vi "State_Machine.vi"(8 "error in (no error)":errorcluster caption="entrée d'erreur (pas d'erreur)", 11 "Get_Voltage en entrée":refnum<class "Zigbee_Reset.lvclass">) -> (0 "error out":errorcluster caption="sortie d'erreur", 2 "Json_String":string, 3 "Get_Voltage en sortie":refnum<class "Zigbee_Reset.lvclass">)   [LabVIEW 2020, in "Library Test.lvlib" / "Zigbee_Reset.lvclass"]
uses:
  Zigbee_Reset.lvclass
  C:/Users/ngarcin/OneDrive - Altyor/Standard TB/Class/Test/Zigbee_Send_Command_UART/Zigbee_Send_Command_UART.lvclass
  C:/Users/ngarcin/OneDrive - Altyor/Standard TB/Class/Test/Test (Default)/Test (Default).lvclass
  Zigbee_Send_Command_UART/Zigbee_Send_Command_UART.lvclass
  Zigbee_Reset.lvclass/Zigbee_Reset.ctl
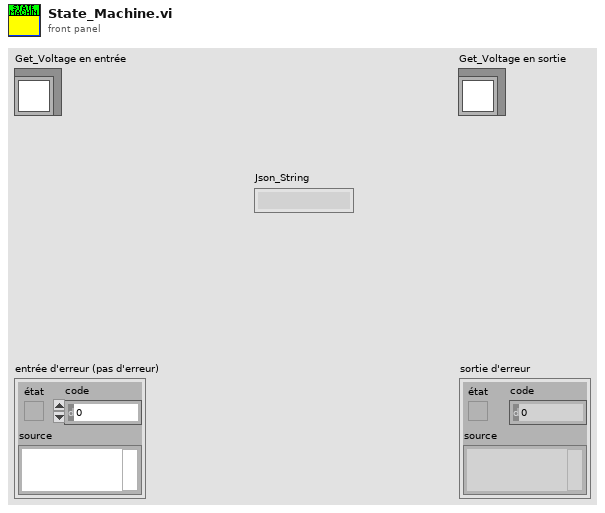
[diagram p1: front panel]
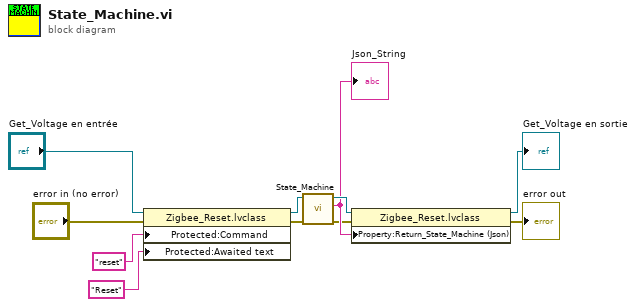
[diagram p0: block diagram]
diagram:
  n1 = property class="Zigbee_Reset.lvclass"(reference="Get_Voltage en entrée", error in="error in (no error)", "Protected:Command"="reset" ("Command"), "Protected:Awaited text"="Reset" ("Awaited text")) -> (reference out=w11:refnum<class "Zigbee_Reset.lvclass">, error out=w10:errorcluster)
  n2 = call-parent "State_Machine.vi"("error in (no error)"=w10, "Send_Frame en entrée"=w11) -> ("error out"=w2:errorcluster, "Json_String"=w4:string, "Send_Frame en sortie"=w5:refnum<class "Zigbee_Reset.lvclass">)  [unwired: 7 in]
  "Json_String" <- w4
  n3 = property class="Zigbee_Reset.lvclass"(reference=w5, error in=w2, "Property:Return_State_Machine (Json)"=w4) -> (reference out=→"Get_Voltage en sortie":refnum<class "Zigbee_Reset.lvclass">, error out=→"error out":errorcluster)
